vi "Messwert im Null-Bereich.vi"(8 "Nullabweichung absolut":dbl, 11 "Messwert":dbl) -> (0 "im Bereich":bool)   [LabVIEW 2020, in "FT-IR.lvlib"]
uses:
  FT-IR.lvlib
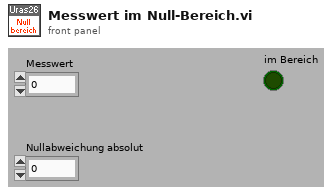
[diagram p1: front panel]
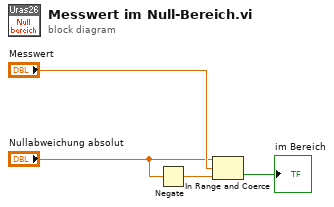
[diagram p0: block diagram]
diagram:
  n1 = Negate(x="Nullabweichung absolut") -> (-x=w2:dbl)
  n2 = In Range and Coerce(upper limit="Nullabweichung absolut", x="Messwert", lower limit=w2) -> (In Range?=→"im Bereich":bool)  [unwired: 1 out]
